vi "I2C Read.vi"(5 "EOF":T1, 6 "Timeout (1000 ms)":u16=1000, 7 "I2C Channel":u8, 8 "Error In":errorcluster, 9 "Bytes To Read":u8, 10 "I2C Slave Address (0)":u8, 11 "LINX Resource":T2) -> (0 "Error Out":errorcluster, 2 "Data":u8[](array[numeric]), 3 "LINX Resource":T2)   [LabVIEW 2020, in "LMH-LINX.lvlib"]
doc: "Read the specified number of bytes from the I2C slave on the specified channel."
uses:
  LMH-LINX.lvlib
  Private/Type Defs/LINX Ref.ctl
  Private/Type Defs/Platform.ctl
  Private/Type Defs/Interface.ctl
  Private/Device/Type Defs/LINX Device Config.ctl
  Private/Device/Type Defs/TCP Config.ctl
  Private/Device/Type Defs/Channels.ctl
  Private/Type Defs/Peripherals/I2C/EOF.ctl
  Private/Type Defs/Peripheral.ctl
  Private/Utilties/Generate Error.vi
  Private/Device/Device.lvlib
  Private/Local IO/Local IO.lvlib
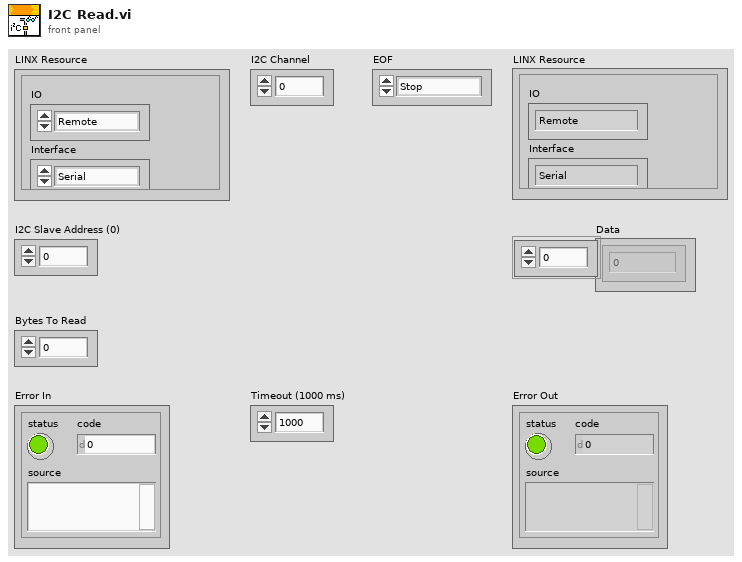
[diagram p1: front panel]
types:
  T1 = typedef "LMH-LINX.lvlib/EOF.ctl" = enum8{"Stop", "Restart", "Restart No Stop", "No Stop"}
  T2 = typedef "LMH-LINX.lvlib/LINX Ref.ctl" = cluster{"IO":T3, "Interface":T4, "LINX Device Config":T5}
  T3 = typedef "LMH-LINX.lvlib/Platform.ctl" = enum16{"Remote", "Local"}
  T4 = typedef "LMH-LINX.lvlib/Interface.ctl" = enum16{"Serial", "TCP"}
  T5 = typedef "LMH-LINX.lvlib/Device.lvlib/LINX Device Config.ctl" = cluster{"Interface":T4, "COM Port":refnum<visa-resource-name>, "TCP Configuration":T6, "Device Family":u8, "Device ID":u8, "Device Name":string, "TCP Ref":refnum<k5>, "Channels":T7}
  T6 = typedef "LMH-LINX.lvlib/Device.lvlib/TCP Config.ctl" = cluster{"IP Address":string, "Port":u16}
  T7 = typedef "LMH-LINX.lvlib/Channels.ctl" = cluster{"DI":u8[], "DO":u8[], "AI":u8[], "AO":u8[], "PWM":u8[], "QE":u8[], "UART":u8[], "I2C 2":u8[], "SPI":u8[], "CAN":u8[], "Servo":u8[], "AI Ref (V)":dbl, "AI Resolution (Bits)":u8, "AO Ref (V)":dbl, "AO Resolution (Bits)":u8}
  T8 = typedef "LMH-LINX.lvlib/Peripheral.ctl" = enum8{"DI", "DO", "AI", "AO", "PWM", "QE", "UART", "I2C", "SPI", "CAN", "Servo"}
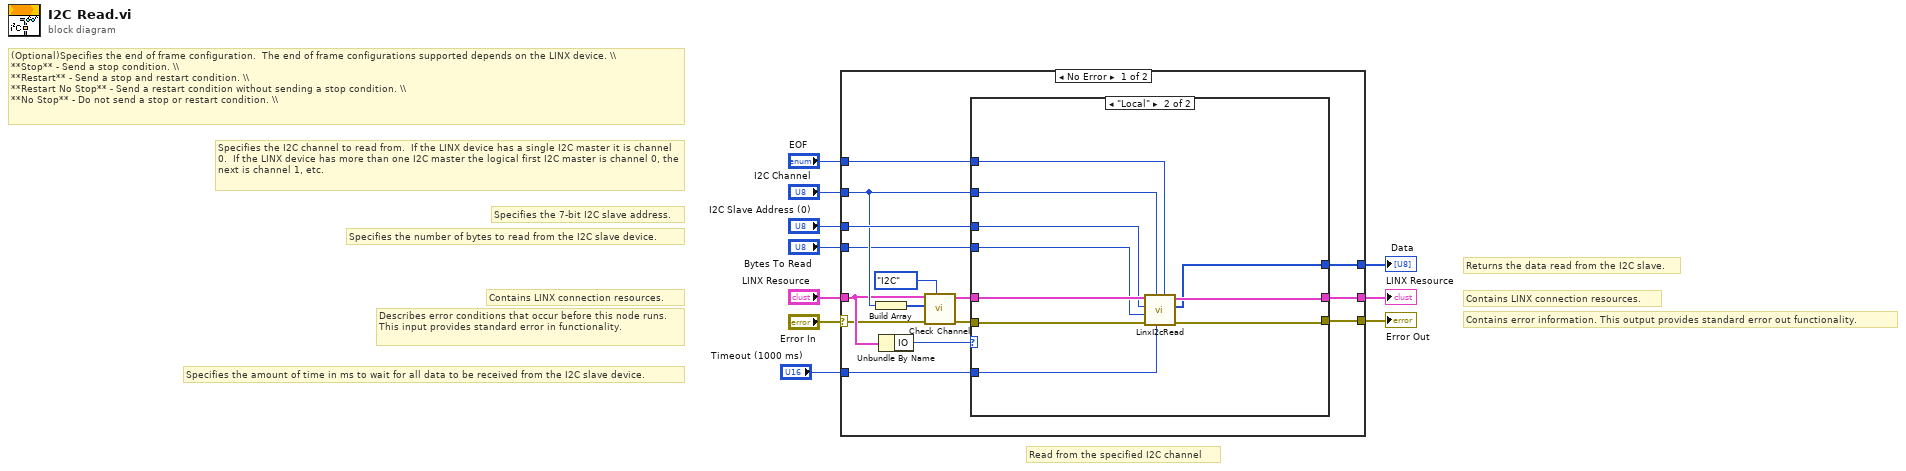
[diagram p0: block diagram]
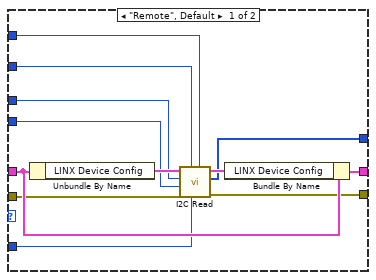
[diagram p2: hidden frame]
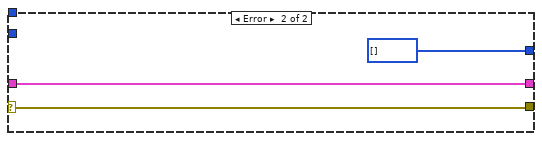
[diagram p3: hidden frame]
diagram:
  # "Specifies the number of bytes to read from the I2C slave device."
  # "Specifies the 7-bit I2C slave address."
  # "(Optional)Specifies the end of frame configuration.  The end of frame configurations supported depends on the LINX device. \\\\ \n**Stop** - Send a stop condition. \\\\ \n**Restart** - Send a stop and restart condition. \\\\\n**Restart No Stop** - Send a restart condition without sending a stop condition. \\\\ \n**No Stop** - Do not send a stop or restart condition. \\\\"
  # "Specifies the amount of time in ms to wait for all data to be received from the I2C slave device."
  # "Returns the data read from the I2C slave."
  # "Specifies the I2C channel to read from.  If the LINX device has a single I2C master it is channel 0.  If the LINX device has more than one I2C master the logical first I2C master is channel 0, the next is channel 1, etc."
  # "Contains LINX connection resources."
  # "Contains error information. This output provides standard error out functionality."
  # "Contains LINX connection resources."
  # "Describes error conditions that occur before this node runs. This input provides standard error in functionality."
  # "Read from the specified I2C channel"
  n1 = case shown="No Error" "Error In" {
    selector: "Error In" -> [w11 w50]
    tunnel: [w24 w50] -> w10
    tunnel: [w23 w49] -> w9
    tunnel: "I2C Slave Address (0)" -> [w22 _]
    tunnel: "I2C Channel" -> [w19 _]
    tunnel: "LINX Resource" -> [w17 w49]
    tunnel: "Bytes To Read" -> [w15 _]
    tunnel: [w14 u8[] [] ("Bytes Read")] -> w4
    tunnel: "Timeout (1000 ms)" -> [w13 _]
    tunnel: "EOF" -> [w12 _]
    frame No Error {
      n2 = Build Array(w19) -> (w18:u8[])
      n3 = Unbundle By Name(w17) -> ("IO"=w25:T3)
      n4 = call "Check Channel.vi"("Peripheral"=Peripheral."I2C", "Error In"=w11, "Channels"=w18, "LINX Resource"=w17) -> ("Error Out"=w20:errorcluster, "LINX Resource"=w16:T2)  [unwired: 5 in, 1 out]
      n5 = case shown="\"Local\"" w25 {
        tunnel: w20 -> [w33 w47]
        tunnel: w16 -> [w37 w46]
        tunnel: [w32 w44] -> w24
        tunnel: [w36 w45] -> w23
        tunnel: w19 -> [w31 w42]
        tunnel: w22 -> [w30 w40]
        tunnel: w15 -> [w29 w38]
        tunnel: [w28 w43] -> w14
        tunnel: w13 -> [w27 w39]
        tunnel: w12 -> [w26 w41]
        frame "Remote", Default {
          n6 = Unbundle By Name(w37) -> ("LINX Device Config"=w35:T5)
          n7 = call "I2C Read.vi"("EOF"=w26, "Timeout (1000 ms)"=w27, "I2C Channel (0)"=w31, "Error In"=w33, "Bytes To Read"=w29, "I2C Slave Address"=w30, "LINX Device Config"=w35) -> ("Error Out"=w32:errorcluster, "Data"=w28:u8[], "LINX Device Config"=w34:T5)  [unwired: 2 in]
          n8 = Bundle By Name(cluster=w37, "LINX Device Config"=w34) -> (w36:T2)
        }
        frame "Local" {
          n9 = call "LinxI2cRead.vi"("EOF"=w41, "Timeout (1000 ms)"=w39, "I2C Channel"=w42, "Error In"=w47, "Num Bytes"=w38, "Slave Address"=w40, "LINX Resource"=w46) -> ("Error Out"=w44:errorcluster, "Data"=w43:u8[], "LINX Resource"=w45:T2)  [unwired: 2 in]
        }
      }
    }
    frame Error {
    }
  }
  "Error Out" <- w10
  "LINX Resource" <- w9
  "Data" <- w4
